vi "Memory (DBL Array).vi"(2 "initialize":bool, 3 "Initial Conditions":dbl[](array[numeric]) format="%.2f", 5 "Input Points":dbl[](array[numeric]) format="%.2f") -> (1 "Output Points":dbl[](array[numeric]) format="%.2f")   [LabVIEW 2017, in "NI_AdvCtrl_nonlinear.lvlib"]
doc: "LabVIEW no longer supports this VI. You can obtain similar functionality by installing the LabVIEW Simulation Module.\n\nStores the input value. It is output(n)=input(n-1), where output(0)=initial condition."
uses:
  <vilib>/addons/control/advanced/NI_AdvCtrl_nonlinear.lvlib
  <vilib>/addons/control/advanced/NI_AdvCtrl_continuous linear.lvlib
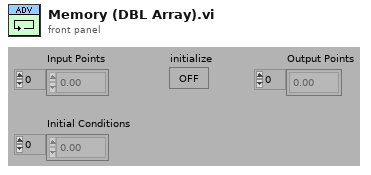
[diagram p1: front panel]
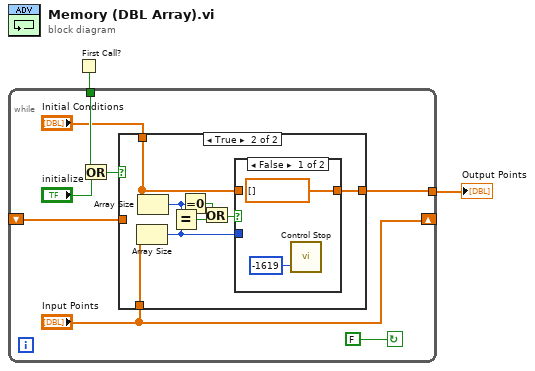
[diagram p0: block diagram]
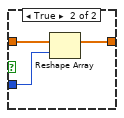
[diagram p3: hidden frame]
diagram:
  n1 = First Call?() -> (First Call?: T/F=w2:bool)
  n2 = while {
    tunnel: w2 -> [w5]
    tunnel: [w10] -> w1
    shift-left: _ -> [w9]
    shift-right: ["Input Points"] -> _
    stop <- FALSE continue-if-true
    n3 = Or(x=w5, y="initialize") -> (x .or. y?=w7:bool)
    n4 = case shown="True" w7 {
      tunnel: [w11 w19] -> w10
      tunnel: w9 -> [w11 _]
      tunnel: "Initial Conditions" -> [_ w17]
      tunnel: "Input Points" -> [_ w16]
      frame False {
      }
      frame True {
        n5 = Array Size(array=w16) -> (size(s)=w12:i32)
        n6 = Array Size(array=w17) -> (size(s)=w14:i32)
        n7 = Equal?(x=w14, y=w12) -> (x = y?=w18:bool)
        n8 = Equal To 0?(x=w14) -> (x = 0?=w13:bool)
        n9 = Or(x=w13, y=w18) -> (x .or. y?=w15:bool)
        n10 = case shown="False" w15 {
          tunnel: w17 -> [_ w24]
          tunnel: [dbl[] [] ("Initial Conditions") w23] -> w19
          tunnel: w12 -> [_ w22]
          frame False {
            n11 = call <vilib>:"Control Stop.vi"("error"=-1619) -> ()  [unwired: 2 out]
          }
          frame True {
            n12 = Reshape Array(w24, w22) -> (w23:dbl[])
          }
        }
      }
    }
  }
  "Output Points" <- w1
